vi "Horner.vi"(10 "Meilleure poly":sgl[](array[numeric]), 11 "X":sgl[](array[numeric])) -> (3 "Y":sgl[](array[numeric]))   [LabVIEW 2013]
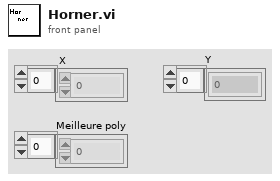
[diagram p1: front panel]
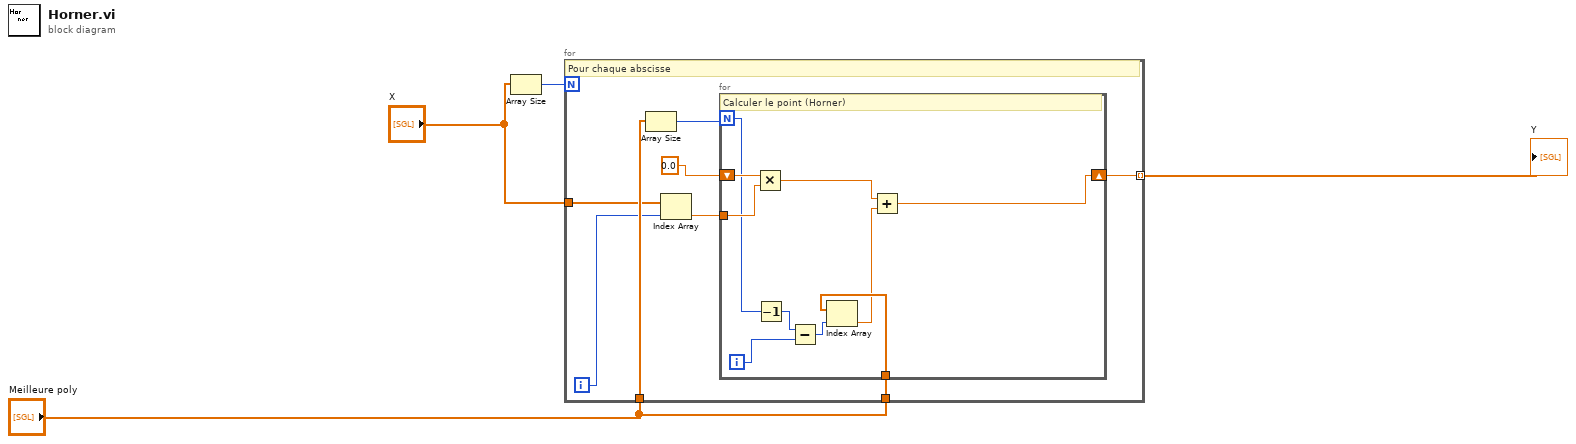
[diagram p0: block diagram]
diagram:
  n1 = Array Size(array="X") -> (size(s)=w1:i32)
  n2 = for {
    N: w1 -> [_]
    tunnel: "Meilleure poly" -> [w11]
    tunnel: "X" -> [w9]
    tunnel: "Meilleure poly" -> [w6]
    tunnel: [w5] -> w3 mode=indexing
    i -> [w10]
    # "Pour chaque abscisse"
    n3 = Array Size(array=w11) -> (size(s)=w12:i32)
    n4 = Index Array(array=w9, index=w10) -> (element=w7:sgl)
    n5 = for {
      N: w12 -> [w18]
      tunnel: w7 -> [w21]
      shift-right: [w13] -> w5
      shift-left: sgl 0.0 -> [w22]
      tunnel: w6 -> [w16]
      i -> [w19]
      # "Calculer le point (Horner)"
      n6 = Multiply(x=w22, y=w21) -> (x*y=w15:sgl)
      n7 = Decrement(x=w18) -> (x-1=w20:i32)
      n8 = Subtract(x=w20, y=w19) -> (x-y=w17:i32)
      n9 = Index Array(array=w16, index=w17) -> (element=w14:sgl)
      n10 = Add(x=w15, y=w14) -> (x+y=w13:sgl)
    }
  }
  "Y" <- w3
